vi "GF_init.vi"(7 "modIdTag":string="F1", 8 "error in (no error)":errorcluster, 11 "channel":refnum<k24>) -> (0 "error out":errorcluster)   [LabVIEW 2021]
uses:
  D:/psychometric_function_v2/lib/Grpc.Core.dll
  lib/Grpc.Core.dll
  D:/psychometric_function_v2/lib/FossilProtosSharp.dll
  lib/FossilProtosSharp.dll
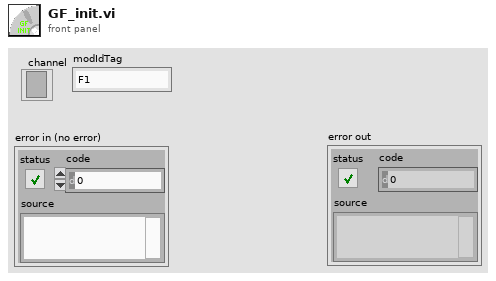
[diagram p1: front panel]
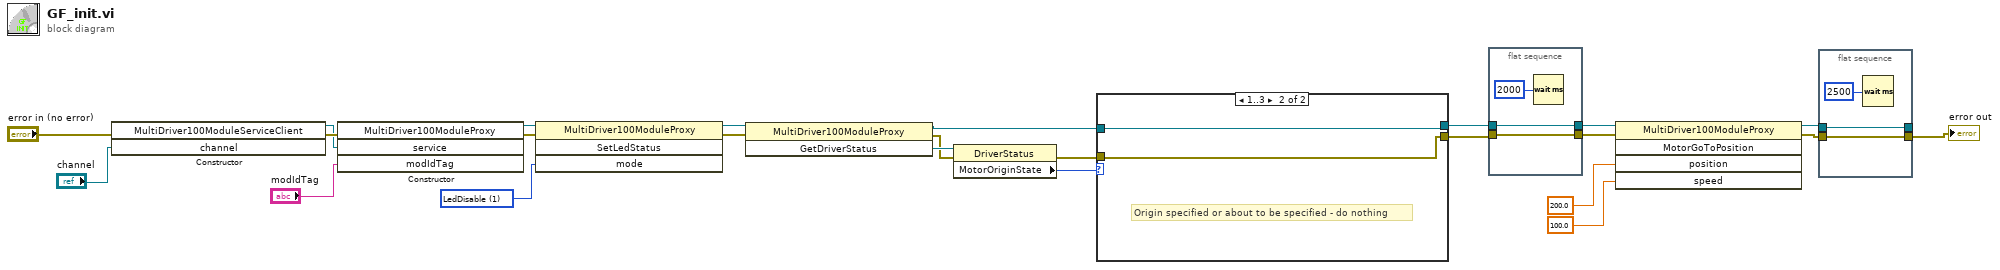
[diagram p0: block diagram]
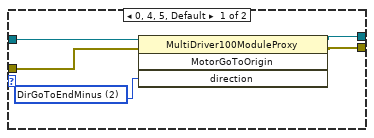
[diagram p2: hidden frame]
diagram:
  w17 = 1 items=["LedUnspecified", "LedDisable", "LedEnable", "LedOnlyErrors", "LedStatus"] ("mode")
  n1 = constructor class="MultiDriver100ModuleServiceClie"(error in="error in (no error)", "channel"="channel") -> (reference out=w18:refnum<k24>, error out=w19:errorcluster)  [unwired: 2 in, 2 out]
  n2 = constructor class="MultiDriver100ModuleProxy"(error in=w19, "service"=w18, "modIdTag"="modIdTag") -> (reference out=w21:refnum<k24>, error out=w20:errorcluster)  [unwired: 2 in, 3 out]
  n3 = invoke class="MultiDriver100ModuleProxy" method="SetLedStatus"(reference=w21, error in=w20, "mode"=w17) -> (reference out=w9:refnum<k24>, error out=w8:errorcluster)  [unwired: 1 in, 2 out]
  n4 = invoke class="MultiDriver100ModuleProxy" method="GetDriverStatus"(reference=w9, error in=w8) -> (reference out=w3:refnum<k24>, error out=w6:errorcluster, "GetDriverStatus"=w7:refnum<k24>)  [unwired: 1 in]
  n5 = property class="DriverStatus"(reference=w7, error in=w6) -> (error out=w4:errorcluster, "MotorOriginState"=w5:i32)  [unwired: 1 out]
  n6 = case shown="1..3" w5 {
    tunnel: w4 -> [w28 w30]
    tunnel: w3 -> [w27 w31]
    tunnel: [w26 w30] -> w2
    tunnel: [w25 w31] -> w1
    frame 0, 4, 5, Default {
      w29 = 2 items=["DirUnspecified", "DirGoToEndPlus", "DirGoToEndMinus"] ("direction")
      n7 = invoke class="MultiDriver100ModuleProxy" method="MotorGoToOrigin"(reference=w27, error in=w28, "direction"=w29) -> (reference out=w25:refnum<k24>, error out=w26:errorcluster)  [unwired: 1 in, 2 out]
    }
    frame 1..3 {
      # "Origin specified or about to be specified - do nothing"
    }
  }
  n8 = flat-sequence {
    tunnel: [w34] -> w14
    tunnel: w1 -> [w34]
    tunnel: w2 -> [w33]
    tunnel: [w33] -> w13
    frame #0 {
      n9 = Wait (ms)(milliseconds to wait=u32 2000) -> ()  [unwired: 1 out]
    }
  }
  n10 = invoke class="MultiDriver100ModuleProxy" method="MotorGoToPosition"(reference=w14, error in=w13, "position"=sgl 200.0, "speed"=sgl 100.0) -> (reference out=w12:refnum<k24>, error out=w11:errorcluster)  [unwired: 1 in, 3 out]
  n11 = flat-sequence {
    tunnel: [w37] -> _
    tunnel: w12 -> [w37]
    tunnel: w11 -> [w36]
    tunnel: [w36] -> w10
    frame #0 {
      n12 = Wait (ms)(milliseconds to wait=u32 2500) -> ()  [unwired: 1 out]
    }
  }
  "error out" <- w10
